vi "VI-Add Override.vi"(0 "LVClassLibrary in":refnum<vi>, 2 "application refnum":refnum<vi>, 7 "Method":string, 9 "Base class":bool, 11 "error in (no error)":errorcluster) -> (4 "reference out":refnum<vi>, 8 "file path":path, 15 "error out":errorcluster)   [LabVIEW 2020]
uses:
  <vilib>/Utility/traverseref.llb/TRef TravTarget.ctl
  <vilib>/Utility/traverseref.llb/VI Scripting - Traverse.lvlib
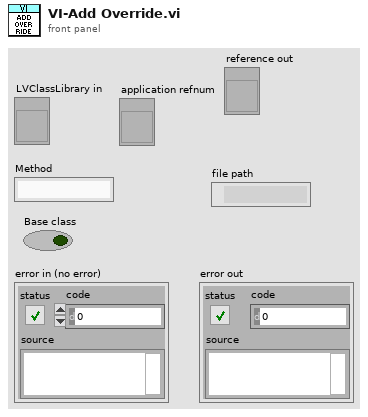
[diagram p1: front panel]
types:
  T1 = typedef "TRef TravTarget.ctl" = enum16{"FP", "BD", "Other"}
  T2 = enum32{"invalid VI type", "Standard VI", "Control VI", "Global VI", "Polymorphic VI", "Configuration VI", "SubSystem", "Facade VI", "Method VI", "Statechart Diagram VI"}
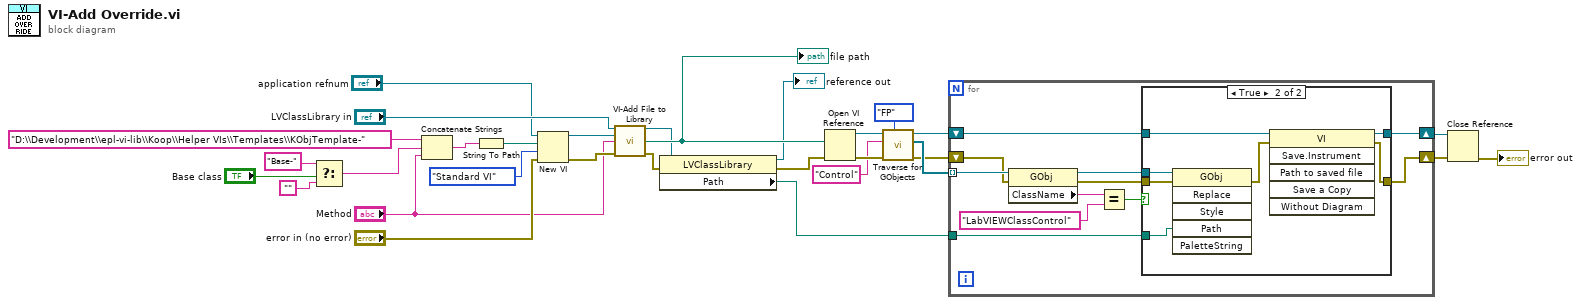
[diagram p0: block diagram]
diagram:
  n1 = Select(t="Base-", s="Base class", f="") -> (s? t:f=w5:string)
  n2 = Concatenate Strings("D:\\Development\\epl-vi-lib\\Koop\\Helper VIs\\Templates\\KObjTemplate-" ("template"), w5, "Method") -> (w25:string)
  n3 = String To Path(string=w25) -> (path=w17:path)
  n4 = New VI(8:"error in (no error)", 9:T2."Standard VI" ("vi type (standard vi)"), 10:w17, 11:"application refnum") -> (0:w28:errorcluster, 3:w29:refnum<vi>)  [unwired: 3 in]
  n5 = call "VI-Add File to Library.vi"("LVClass.Create in"="LVClassLibrary in", "VI ref"=w29, "Filename"="Method", "error in (no error)"=w28) -> ("reference out"=w9:refnum<vi>, "file path"=w23:path, "error out"=w8:errorcluster)  [unwired: 9 in]
  "file path" <- w23
  n6 = property class="LVClassLibrary"(reference=w9, error in=w8) -> (reference out=→"reference out":refnum<vi>, error out=w7:errorcluster, "Path"=w14:path)
  n7 = Open VI Reference(vi path=w23, error in (no error)=w7) -> (vi reference=w22:refnum<vi>, error out=w21:errorcluster)  [unwired: 4 in]
  n8 = call <vilib>:"Traverse for GObjects.vi"("Traverse Target"=TRef_TravTarget."FP", "error in (no error)"=w21, "Class Name"="Control", "VI Refnum"=w22) -> ("error out"=w16:errorcluster, "References"=w18:refnum<vi>[], "dup VI Refnum"=w11:refnum<vi>)  [unwired: 4 in, 1 out]
  n9 = for {
    tunnel: w18 -> [w41] mode=indexing
    shift-right: [w34] -> w13
    shift-left: w16 -> [w40]
    tunnel: w14 -> [w33]
    shift-right: [w31] -> w10
    shift-left: w11 -> [w32]
    n10 = property class="GObj"(reference=w41, error in=w40) -> (reference out=w37:refnum<vi>, error out=w35:errorcluster, "ClassName"=w39:string)
    n11 = Equal?(x=w39, y="LabVIEWClassControl") -> (x = y?=w36:bool)
    n12 = case shown="True" w36 {
      tunnel: w37 -> [_ w50]
      tunnel: w35 -> [w43 w49]
      tunnel: [w43 w45] -> w34
      tunnel: w33 -> [_ w48]
      tunnel: w32 -> [w42 w47]
      tunnel: [w42 w44] -> w31
      frame False {
      }
      frame True {
        n13 = invoke class="GObj" method="Replace"(reference=w50, error in=w49, "Path"=w48) -> (error out=w46:errorcluster)  [unwired: 3 in, 5 out]
        n14 = invoke class="VI" method="Save.Instrument"(reference=w47, error in=w46) -> (reference out=w44:refnum<vi>, error out=w45:errorcluster)  [unwired: 4 in, 4 out]
      }
    }
  }
  n15 = Close Reference(reference=w10, error in (no error)=w13) -> (error out=→"error out":errorcluster)
